vi "sendMessage.vi"(8 "error in (no error)":errorcluster, 10 "message":string, 11 "TCPClient in":refnum<class "TCPClient.lvclass">) -> (0 "error out":errorcluster, 3 "TCPClient out":refnum<class "TCPClient.lvclass">)   [LabVIEW 2016, in "TCPClient.lvclass"]
uses:
  TCPClient.lvclass
  TCPClient.lvclass/TCPClient.ctl
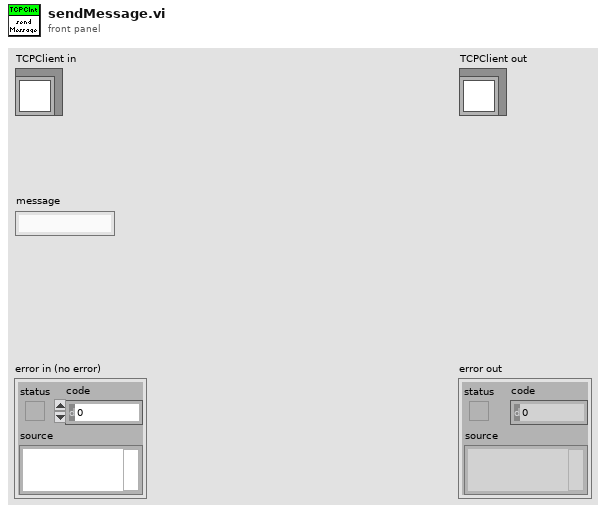
[diagram p1: front panel]
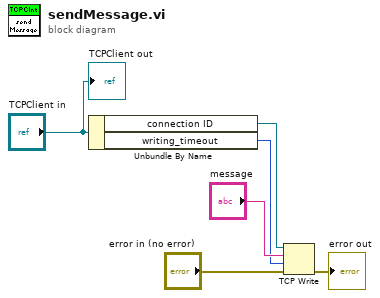
[diagram p0: block diagram]
diagram:
  n1 = Unbundle By Name("TCPClient in") -> ("connection ID"=w2:refnum<k5>, "writing_timeout"=w1:i32)
  n2 = TCP Write(connection ID=w2, data in="message", error in (no error)="error in (no error)", 9:w1) -> (error out=→"error out":errorcluster)  [unwired: 2 out]
  "TCPClient out" <- "TCPClient in"
